vi "Engine Out - Variable Valve Actuation.vi"(6 "Sync":bool, 7 "Cam2 VVT Advance Setpoint [CAD]":sgl format="%.2f", 8 "Cam1 VVT Advance Setpoint [CAD]":sgl format="%.2f", 9 "BattV [V]":sgl, 10 "Control Inputs":T2={"Engine Speed [RPM]"=0.0, "Engine Status"=enum."STALLED", "Load Control \nMode"=enum."Max Speed Governor", "dt(s)"=0.0, "Number of Cylinders"=0, "Engine Displacement [cc]"=0.0, "StoichAFR"=0.0, "Q.LHV Fuel [kJ/kg]"=0.0, "BattV PSU [V]"=0.0, "12V PSU [V]"=0.0, "5V PSU [V]"=0.0, "Pedal Position [%]"=0.0, "Oil Pressure [kPa]"=0.0, "Oil Temp [C]"=0.0, "Oil Level [%]"=0.0, "Engine Coolant Temp (ECT) [C]"=0.0, "Engine Coolant Pressure [kPa]"=0.0, "Rail Pressure [bar]"=0.0, "Fuel Pressure [kPa]"=0.0, "Fuel Temp [C]"=0.0, "Vacuum Pressure [kPa]"=0.0, "Throttle Position [%]"=0.0, "Cam1 Advance [CAD]"=0.0, "Cam2 Advance [CAD]"=0.0, "Cam3 Advance [CAD]"=0.0, "Cam4 Advance [CAD]"=0.0, "CA50 Control Output [CAD]"=[], "CA50 Control Output Valid"=[], "Intake Air Temp (IAT) [C]"=0.0, "Barometric Air Pressure [kPa]"=0.0, "Intake Air Rel. Humidity [%]"=0.0, "Mass Air Flow (MAF) [kg/hr]"=0.0, "Turbo Inlet Air Pressure [kPa]"=0.0, "Turbo Inlet Air Temp [C]"=0.0, "Turbo Outlet Air Pressure [kPa]"=0.0, "Turbo Outlet Air Temp [C]"=0.0, "CAC Outlet Pressure [kPa]"=0.0, "CAC Outlet Temp [C]"=0.0, "Intake Manifold Pressure (MAP) [kPa]"=0.0, "Intake Manifold Temp (MAT) [C]"=0.0, "Exhaust Manifold Pressure [kPa]"=0.0, "Exhaust Manifold Temp [C]"=0.0, "HighP EGR Cooler Outlet Pressure [kPa]"=0.0, "HighP EGR Cooler Outlet Temp [C]"=0.0, "HighP EGR Differential Pressure [kPa]"=0.0, "HighP EGR Valve Position [%]"=0.0, "Turbo Outlet Exhaust Pressure [kPa]"=0.0, "Turbo Outlet Exhaust Temp [C]"=0.0, "VGT Position 1 [%]"=0.0, "VGT Position 2 [%]"=0.0, "Turbo Speed 1 [RPM]"=0.0, "Turbo Speed 2 [RPM]"=0.0, "LowP EGR Differential Pressure [kPa]"=0.0, "LowP EGR Valve Position [%]"=0.0, "UEGO1Lambda"=0.0, "UEGO1_Hot"=FALSE, "UEGO2Lambda"=0.0, "UEGO2_Hot"=FALSE, "Knock Intensity"=[], "Knock"=[]} {"Knock Intensity" format="%.2f"; "CA50 Control Output [CAD]" format="%.2f"; "Exhaust Manifold Temp [C]" format="%#_6f"; "UEGO2Lambda" format="%.2f"; "Intake Manifold Temp (MAT) [C]" format="%#_6f"; "UEGO1Lambda" format="%.2f"}) -> (2 "Cam2 LS Output":T1, 3 "Cam1 LS Output":T1)   [LabVIEW 2015, in "ECS-RT.lvlib"]
uses:
  ECS-RT.lvlib
  Typedefs/Control Inputs/Control Inputs.ctl
  Typedefs/EPT/Engine Status.ctl
  Typedefs/MISC/Load Control Mode.ctl
  Typedefs/Raw Outputs/LS.ctl
  ECS-Shared.lvlib
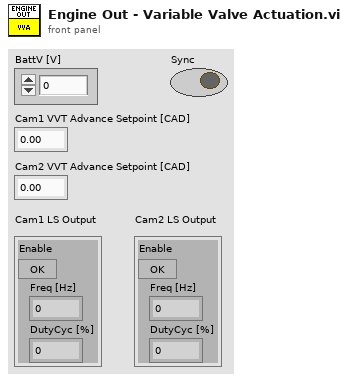
[diagram p1: front panel]
types:
  T1 = typedef "ECS-Shared.lvlib/LS.ctl" = cluster{"Enable":bool, "Freq [Hz]":sgl, "DutyCyc [%]":sgl}
  T2 = typedef "ECS-Shared.lvlib/Control Inputs.ctl" = cluster{"Engine Speed [RPM]":sgl, "Engine Status":T3, "Load Control \nMode":T4, "dt(s)":sgl, "Number of Cylinders":u8, "Engine Displacement [cc]":sgl, "StoichAFR":sgl, "Q.LHV Fuel [kJ/kg]":sgl, "BattV PSU [V]":sgl, "12V PSU [V]":sgl, "5V PSU [V]":sgl, "Pedal Position [%]":sgl, "Oil Pressure [kPa]":sgl, "Oil Temp [C]":sgl, "Oil Level [%]":sgl, "Engine Coolant Temp (ECT) [C]":sgl, "Engine Coolant Pressure [kPa]":sgl, "Rail Pressure [bar]":sgl, "Fuel Pressure [kPa]":sgl, "Fuel Temp [C]":sgl, "Vacuum Pressure [kPa]":sgl, "Throttle Position [%]":sgl, "Cam1 Advance [CAD]":sgl, "Cam2 Advance [CAD]":sgl, "Cam3 Advance [CAD]":sgl, "Cam4 Advance [CAD]":sgl, "CA50 Control Output [CAD]":sgl[], "CA50 Control Output Valid":bool[], "Intake Air Temp (IAT) [C]":sgl, "Barometric Air Pressure [kPa]":sgl, "Intake Air Rel. Humidity [%]":sgl, "Mass Air Flow (MAF) [kg/hr]":sgl, "Turbo Inlet Air Pressure [kPa]":sgl, "Turbo Inlet Air Temp [C]":sgl, "Turbo Outlet Air Pressure [kPa]":sgl, "Turbo Outlet Air Temp [C]":sgl, "CAC Outlet Pressure [kPa]":sgl, "CAC Outlet Temp [C]":sgl, "Intake Manifold Pressure (MAP) [kPa]":sgl, "Intake Manifold Temp (MAT) [C]":sgl, "Exhaust Manifold Pressure [kPa]":sgl, "Exhaust Manifold Temp [C]":sgl, "HighP EGR Cooler Outlet Pressure [kPa]":sgl, "HighP EGR Cooler Outlet Temp [C]":sgl, "HighP EGR Differential Pressure [kPa]":sgl, "HighP EGR Valve Position [%]":sgl, "Turbo Outlet Exhaust Pressure [kPa]":sgl, "Turbo Outlet Exhaust Temp [C]":sgl, "VGT Position 1 [%]":sgl, "VGT Position 2 [%]":sgl, "Turbo Speed 1 [RPM]":sgl, "Turbo Speed 2 [RPM]":sgl, "LowP EGR Differential Pressure [kPa]":sgl, "LowP EGR Valve Position [%]":sgl, "UEGO1Lambda":sgl, "UEGO1_Hot":bool, "UEGO2Lambda":sgl, "UEGO2_Hot":bool, "Knock Intensity":sgl[], "Knock":bool[]}
  T3 = typedef "ECS-Shared.lvlib/Engine Status.ctl" = enum16{"OFF", "STALLED", "CRANKING", "RUNNING", "ACCEL", "DECEL", "SAFE"}
  T4 = typedef "ECS-Shared.lvlib/Load Control Mode.ctl" = enum16{"No Governor", "Min Speed Governor", "Max Speed Governor"}
  T5 = cluster{"PID_Kp":sgl, "PID_Ti":sgl, "PID_Td":sgl, "PID_FF":sgl, "Non-PID_FF":sgl, "PID_Min":sgl, "PID_Max":sgl}
  T6 = cluster{"BattV [V]":sgl, "ValveNominalResitance":sgl, "Min Duty Cycle":sgl, "Manual Max Duty Cycle":sgl, "Manual Duty Cycle":sgl, "Duty Cycle Override":bool, "Drive Frequency":sgl}
  T7 = cluster{"DutyCycle_Output":sgl, "Calculated Max Duty Cycle":sgl, "Valve Current Flow":sgl, "PID_Output":sgl}
  T8 = cluster{"ProportionalAction":sgl, "IntegralAction":sgl, "DerivativeAction":sgl}
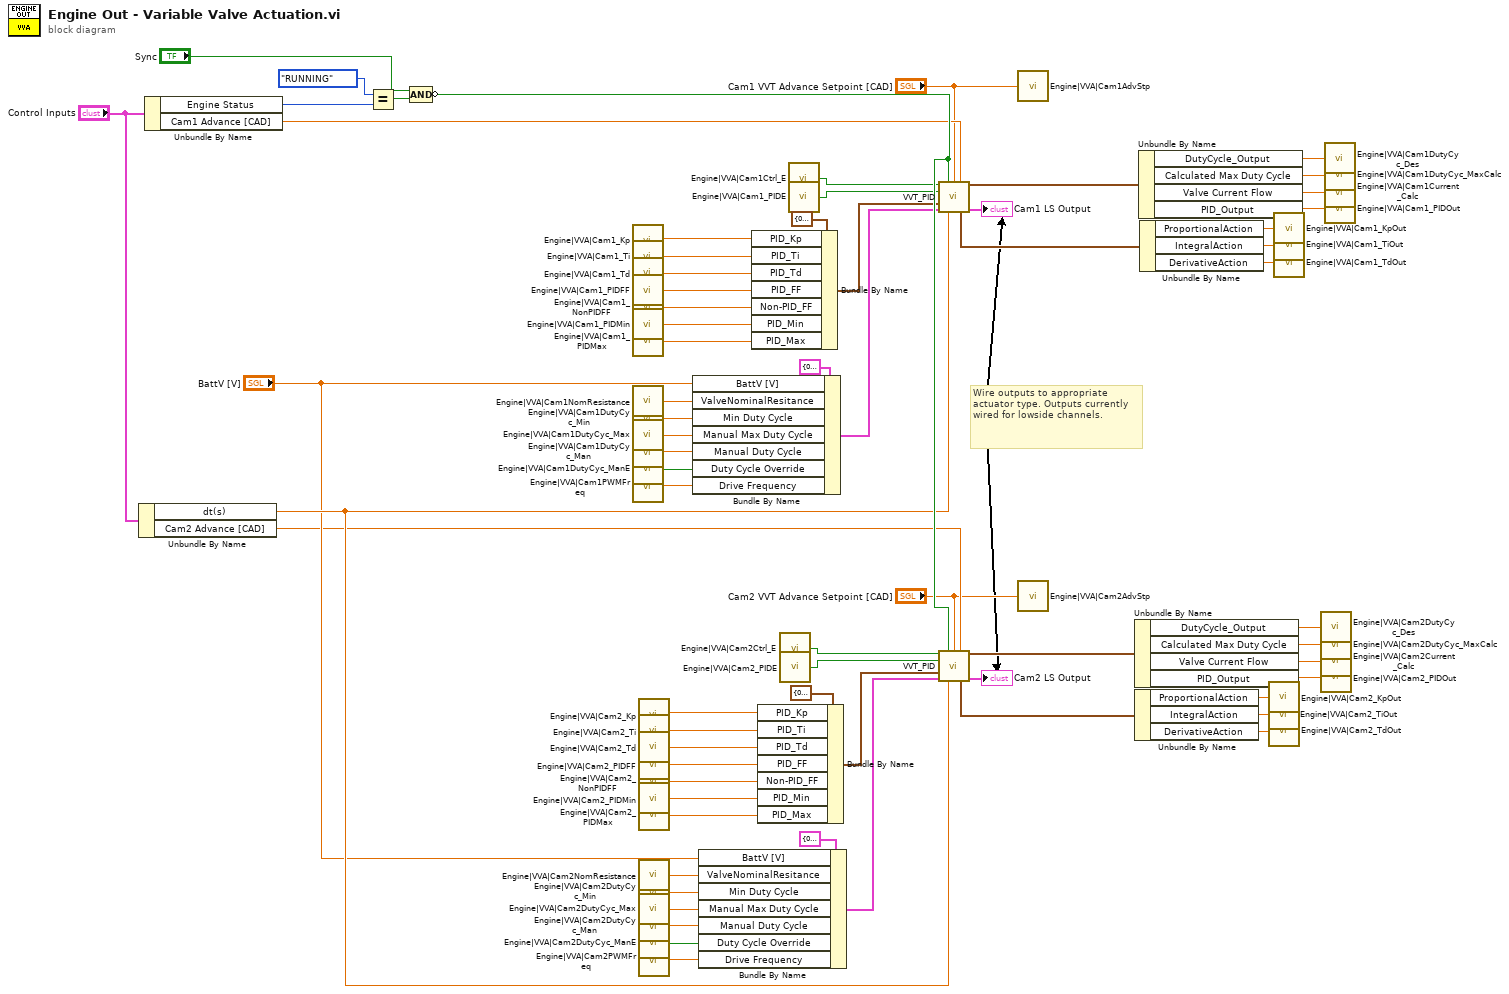
[diagram p0: block diagram]
diagram:
  # "Wire outputs to appropriate actuator type. Outputs currently wired for lowside channels."
  n1 = Unbundle By Name("Control Inputs") -> ("dt(s)"=w14:sgl, "Cam2 Advance [CAD]"=w8:sgl)
  n2 = Unbundle By Name("Control Inputs") -> ("Engine Status"=w41:T3, "Cam1 Advance [CAD]"=w9:sgl)
  n3 = Equal?(x=Engine_Status."RUNNING", y=w41) -> (x = y?=w2:bool)
  n4 = Compound Arithmetic op=AND("Sync", w2) -> (invert w70:bool)
  n5 = call "Engine|VVA|Cam1_Kp"() -> ("Value"=w27:sgl)
  n6 = call "Engine|VVA|Cam1_Ti"() -> ("Value"=w26:sgl)
  n7 = call "Engine|VVA|Cam1_Td"() -> ("Value"=w25:sgl)
  n8 = call "Engine|VVA|Cam1_PIDFF"() -> ("Value"=w24:sgl)
  n9 = call "Engine|VVA|Cam1_NonPIDFF"() -> ("Value"=w23:sgl)
  n10 = call "Engine|VVA|Cam1_PIDMin"() -> ("Value"=w22:sgl)
  n11 = call "Engine|VVA|Cam1_PIDMax"() -> ("Value"=w21:sgl)
  n12 = call "Engine|VVA|Cam1NomResistance"() -> ("Value"=w16:sgl)
  n13 = call "Engine|VVA|Cam1DutyCyc_Min"() -> ("Value"=w17:sgl)
  n14 = call "Engine|VVA|Cam1DutyCyc_Max"() -> ("Value"=w15:sgl)
  n15 = call "Engine|VVA|Cam1DutyCyc_Man"() -> ("Value"=w18:sgl)
  n16 = call "Engine|VVA|Cam1DutyCyc_ManE"() -> ("Value"=w19:bool)
  n17 = call "Engine|VVA|Cam1PWMFreq"() -> ("Value"=w20:sgl)
  n18 = call "Engine|VVA|Cam2_Kp"() -> ("Value"=w63:sgl)
  n19 = call "Engine|VVA|Cam2_Ti"() -> ("Value"=w62:sgl)
  n20 = call "Engine|VVA|Cam2_Td"() -> ("Value"=w61:sgl)
  n21 = call "Engine|VVA|Cam2_PIDFF"() -> ("Value"=w60:sgl)
  n22 = call "Engine|VVA|Cam2_NonPIDFF"() -> ("Value"=w59:sgl)
  n23 = call "Engine|VVA|Cam2_PIDMin"() -> ("Value"=w58:sgl)
  n24 = call "Engine|VVA|Cam2_PIDMax"() -> ("Value"=w57:sgl)
  n25 = call "Engine|VVA|Cam2NomResistance"() -> ("Value"=w52:sgl)
  n26 = call "Engine|VVA|Cam2DutyCyc_Min"() -> ("Value"=w53:sgl)
  n27 = call "Engine|VVA|Cam2DutyCyc_Max"() -> ("Value"=w51:sgl)
  n28 = call "Engine|VVA|Cam2DutyCyc_Man"() -> ("Value"=w54:sgl)
  n29 = call "Engine|VVA|Cam2DutyCyc_ManE"() -> ("Value"=w55:bool)
  n30 = call "Engine|VVA|Cam2PWMFreq"() -> ("Value"=w56:sgl)
  n31 = Bundle By Name(cluster=T6 {"BattV [V]"=0.0, "ValveNominalResitance"=0.0, "Min Duty Cycle"=0.0, "Manual Max Duty Cycle"=0.0, "Manual Duty Cycle"=0.0, "Duty Cycle Override"=FALSE, "Drive Frequency"=0.0} ("Output Management Controls"), "BattV [V]"="BattV [V]", "ValveNominalResitance"=w16, "Min Duty Cycle"=w17, "Manual Max Duty Cycle"=w15, "Manual Duty Cycle"=w18, "Duty Cycle Override"=w19, "Drive Frequency"=w20) -> (w36:T6)
  n32 = Bundle By Name(cluster=T6 {"BattV [V]"=0.0, "ValveNominalResitance"=0.0, "Min Duty Cycle"=0.0, "Manual Max Duty Cycle"=0.0, "Manual Duty Cycle"=0.0, "Duty Cycle Override"=FALSE, "Drive Frequency"=0.0} ("Output Management Controls"), "BattV [V]"="BattV [V]", "ValveNominalResitance"=w52, "Min Duty Cycle"=w53, "Manual Max Duty Cycle"=w51, "Manual Duty Cycle"=w54, "Duty Cycle Override"=w55, "Drive Frequency"=w56) -> (w69:T6)
  n33 = Bundle By Name(cluster=T5 {"PID_Kp"=0.0, "PID_Ti"=0.01, "PID_Td"=0.0, "PID_FF"=0.0, "Non-PID_FF"=0.0, "PID_Min"=-100.0, "PID_Max"=100.0} ("PID Settings"), "PID_Kp"=w27, "PID_Ti"=w26, "PID_Td"=w25, "PID_FF"=w24, "Non-PID_FF"=w23, "PID_Min"=w22, "PID_Max"=w21) -> (w5:T5)
  n34 = Bundle By Name(cluster=T5 {"PID_Kp"=0.0, "PID_Ti"=0.01, "PID_Td"=0.0, "PID_FF"=0.0, "Non-PID_FF"=0.0, "PID_Min"=-100.0, "PID_Max"=100.0} ("PID Settings"), "PID_Kp"=w63, "PID_Ti"=w62, "PID_Td"=w61, "PID_FF"=w60, "Non-PID_FF"=w59, "PID_Min"=w58, "PID_Max"=w57) -> (w68:T5)
  n35 = call "Engine|VVA|Cam2Ctrl_E"() -> ("Value"=w64:bool)
  n36 = call "Engine|VVA|Cam2_PIDE"() -> ("Value"=w65:bool)
  n37 = call "Engine|VVA|Cam1Ctrl_E"() -> ("Value"=w37:bool)
  n38 = call "Engine|VVA|Cam1_PIDE"() -> ("Value"=w38:bool)
  n39 = call "VVT_PID.vi"("Control Enable"=w37, "Fault Input"=w70, "VVT Angle Setpoint"="Cam1 VVT Advance Setpoint [CAD]", "Cam_RisingEdge_Feedback"=w9, "PID Enable"=w38, "PID Settings"=w5, "Output Management Controls"=w36, "dt (s)"=w14) -> ("Output"=w39:T7, "PID_Action_Output"=w40:T8, "LS_Output"=→"Cam1 LS Output":T1)  [unwired: 5 in]
  n40 = call "VVT_PID.vi"("Control Enable"=w64, "Fault Input"=w70, "VVT Angle Setpoint"="Cam2 VVT Advance Setpoint [CAD]", "Cam_RisingEdge_Feedback"=w8, "PID Enable"=w65, "PID Settings"=w68, "Output Management Controls"=w69, "dt (s)"=w14) -> ("Output"=w66:T7, "PID_Action_Output"=w67:T8, "LS_Output"=→"Cam2 LS Output":T1)  [unwired: 5 in]
  n41 = call "Engine|VVA|Cam1AdvStp"("Value"="Cam1 VVT Advance Setpoint [CAD]") -> ()
  n42 = call "Engine|VVA|Cam2AdvStp"("Value"="Cam2 VVT Advance Setpoint [CAD]") -> ()
  n43 = Unbundle By Name(w66) -> ("DutyCycle_Output"=w46:sgl, "Calculated Max Duty Cycle"=w45:sgl, "Valve Current Flow"=w44:sgl, "PID_Output"=w43:sgl)
  n44 = Unbundle By Name(w67) -> ("ProportionalAction"=w47:sgl, "IntegralAction"=w48:sgl, "DerivativeAction"=w49:sgl)
  n45 = Unbundle By Name(w39) -> ("DutyCycle_Output"=w31:sgl, "Calculated Max Duty Cycle"=w30:sgl, "Valve Current Flow"=w29:sgl, "PID_Output"=w28:sgl)
  n46 = Unbundle By Name(w40) -> ("ProportionalAction"=w32:sgl, "IntegralAction"=w33:sgl, "DerivativeAction"=w34:sgl)
  n47 = call "Engine|VVA|Cam2_KpOut"("Value"=w47) -> ()
  n48 = call "Engine|VVA|Cam2_TiOut"("Value"=w48) -> ()
  n49 = call "Engine|VVA|Cam2_TdOut"("Value"=w49) -> ()
  n50 = call "Engine|VVA|Cam1_KpOut"("Value"=w32) -> ()
  n51 = call "Engine|VVA|Cam1_TiOut"("Value"=w33) -> ()
  n52 = call "Engine|VVA|Cam1_TdOut"("Value"=w34) -> ()
  n53 = call "Engine|VVA|Cam2DutyCyc_Des"("Value"=w46) -> ()
  n54 = call "Engine|VVA|Cam2DutyCyc_MaxCalc"("Value"=w45) -> ()
  n55 = call "Engine|VVA|Cam2Current_Calc"("Value"=w44) -> ()
  n56 = call "Engine|VVA|Cam2_PIDOut"("Value"=w43) -> ()
  n57 = call "Engine|VVA|Cam1DutyCyc_Des"("Value"=w31) -> ()
  n58 = call "Engine|VVA|Cam1DutyCyc_MaxCalc"("Value"=w30) -> ()
  n59 = call "Engine|VVA|Cam1Current_Calc"("Value"=w29) -> ()
  n60 = call "Engine|VVA|Cam1_PIDOut"("Value"=w28) -> ()
